vi "lidar pulse wrapper.vi"(11 "VISA resource name":refnum<visa-resource-name>) -> (1 "Angle Array":dbl[](array[numeric]), 2 "Distance Array":u32[](array[numeric]), 3 "VISA resource name out":refnum<visa-resource-name>)   [LabVIEW 2017]
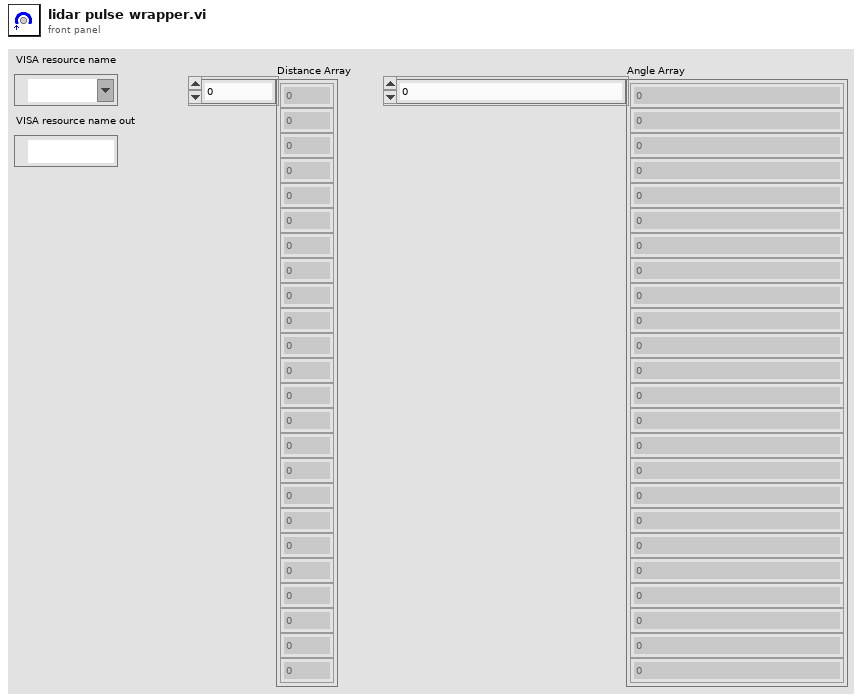
[diagram p1: front panel]
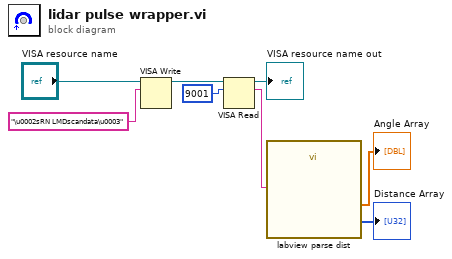
[diagram p0: block diagram]
diagram:
  n1 = VISA Write(VISA resource name="VISA resource name", write buffer="\u0002sRN LMDscandata\u0003") -> (VISA resource name out=w6:refnum<visa-resource-name>)  [unwired: 1 in, 2 out]
  n2 = VISA Read(VISA resource name=w6, byte count=u32 9001) -> (VISA resource name out=→"VISA resource name out":refnum<visa-resource-name>, read buffer=w8:string)  [unwired: 1 in, 2 out]
  n3 = call "labview parse dist.vi"("Telegram String"=w8) -> ("Angle Array"=→"Angle Array":dbl[], "Distance Array"=→"Distance Array":u32[])  [unwired: 8 in]
